vi "Reset Pin Names.vi"(0 "Display State In":T1, 7 "Connector":string="roboRIO Connector SPI", 9 "Container State":T2, 11 "error in (no error)":errorcluster) -> (4 "Display State Out":T1, 15 "error out":errorcluster)   [LabVIEW 2021, in "roboRIO SPI.xctl"]
uses:
  <vilib>/myRIO/Common/Instrument Driver Framework/Utilities/xctls/roboRIO SPI/roboRIO SPI.xctl
  <vilib>/_xctls/Container State.ctl
  <vilib>/myRIO/Common/Instrument Driver Framework/Utilities/xctls/roboRIO SPI/State.ctl
  <vilib>/myRIO/Common/Instrument Driver Framework/Utilities/xctls/utilities/vis/myRIOXC Read Pin Name.vi
  <vilib>/_xctls/XControlSupport.lvlib
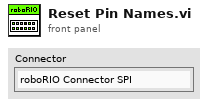
[diagram p1: front panel]
types:
  T1 = typedef "roboRIO SPI.xctl/State.ctl" = cluster{"Pin Disabled?":enum8{"Enabled", "Disabled", "Disabled and Grayed Out"}[], "Pin Name":string[]}
  T2 = typedef "XControlSupport.lvlib/Container State.ctl" = cluster{"Indicator?":bool, "Run Mode?":bool, " Refnum":refnum<vi>}
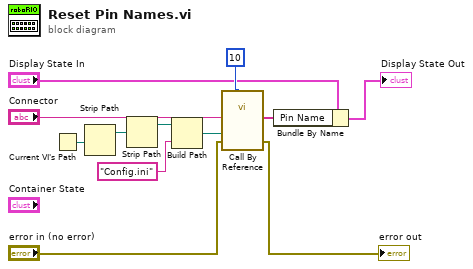
[diagram p0: block diagram]
diagram:
  n1 = Current VI's Path() -> (path=w8:path)
  n2 = Strip Path(path=w8) -> (stripped path=w10:path)  [unwired: 1 out]
  n3 = Strip Path(path=w10) -> (stripped path=w11:path)  [unwired: 1 out]
  n4 = Build Path(base path=w11, name or relative path="Config.ini") -> (appended path=w12:path)
  n5 = call-by-ref "?"("Size"=10, "error in"="error in (no error)", "Path"=w12, "Connector"="Connector") -> ("error out"=→"error out":errorcluster, "Default Names"=w3:string[])  [unwired: 8 in, 2 out]
  n6 = Bundle By Name(cluster="Display State In", "Pin Name"=w3) -> (→"Display State Out":T1)
